vi "Keysight 34401A Get Session.vi"(7 "operation":enum16{"Get Session", "Close Session"}(ring), 8 "error in (no error)":errorcluster, 9 "Reset (True)":bool=TRUE, 10 "ID Query (True)":bool=TRUE, 11 "VISA resource name":refnum<visa-resource-name>) -> (0 "error out":errorcluster, 3 "VISA resource name out":refnum<visa-resource-name>)   [LabVIEW 2020, in "Keysight 34401A DMM Measurement.lvlib"]
uses:
  Keysight 34401A DMM Measurement.lvlib
  <instrlib>/Agilent 34401/Agilent 34401.lvlib
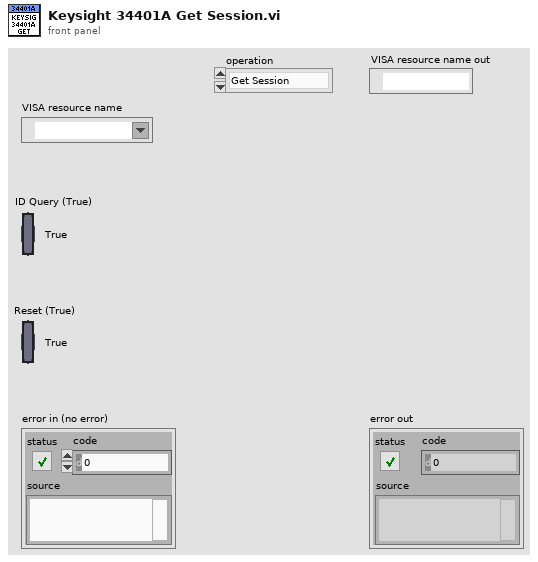
[diagram p1: front panel]
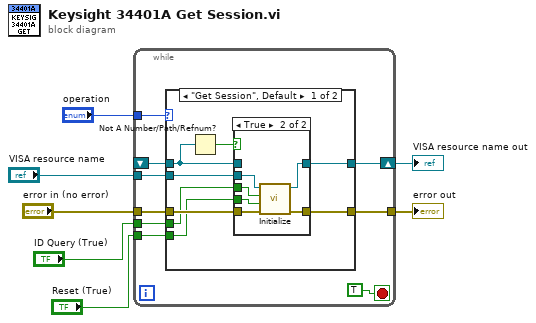
[diagram p0: block diagram]
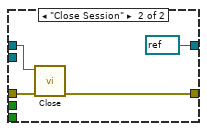
[diagram p3: hidden frame]
diagram:
  n1 = while {
    tunnel: "operation" -> [w16]
    shift-right: [w15] -> w6
    shift-left: _ -> [w14]
    tunnel: [w13] -> w5
    tunnel: "error in (no error)" -> [w11]
    tunnel: "Reset (True)" -> [w10]
    tunnel: "ID Query (True)" -> [w9]
    tunnel: "VISA resource name" -> [w8]
    stop <- TRUE stop-if-true
    n2 = case shown="\"Get Session\", Default" w16 {
      tunnel: [w24 refnum<visa-resource-name> refnum ("VISA resource name out")] -> w15
      tunnel: w14 -> [w17 w35]
      tunnel: [w22 w34] -> w13
      tunnel: w11 -> [w21 w36]
      tunnel: w10 -> [w20 _]
      tunnel: w9 -> [w19 _]
      tunnel: w8 -> [w18 _]
      frame "Get Session", Default {
        n3 = Not A Number/Path/Refnum?(number/path/refnum=w17) -> (NaN/Path/Refnum?=w23:bool)
        n4 = case shown="True" w23 {
          tunnel: [w26 w32] -> w24
          tunnel: [w25 w31] -> w22
          tunnel: w21 -> [w25 w30]
          tunnel: w20 -> [_ w29]
          tunnel: w19 -> [_ w28]
          tunnel: w18 -> [_ w27]
          tunnel: w17 -> [w26 _]
          frame False {
          }
          frame True {
            n5 = call <instrlib>:"Initialize.vi"("error in (no error)"=w30, "Reset (True)"=w29, "ID Query (True)"=w28, "VISA resource name"=w27) -> ("error out"=w31:errorcluster, "VISA resource name out"=w32:refnum<visa-resource-name>)  [unwired: 6 in]
          }
        }
      }
      frame "Close Session" {
        n6 = call <instrlib>:"Close.vi"("error in (no error)"=w36, "VISA resource name"=w35) -> ("error out"=w34:errorcluster)  [unwired: 9 in]
      }
    }
  }
  "error out" <- w5
  "VISA resource name out" <- w6
